vi "Read Props.vi"(8 "error in (no error)":errorcluster, 11 "VerticalSliderControlEditorPanel in":refnum<class "VerticalSliderControlEditorPanel.lvclass">) -> (0 "error out":errorcluster, 2 "Props":T1, 3 "VerticalSliderControlEditorPanel out":refnum<class "VerticalSliderControlEditorPanel.lvclass">)   [LabVIEW 2020, in "VolatusGUIControls.lvlib" / "VerticalSliderControlEditorPanel.lvclass"]
uses:
  VerticalSliderControlEditorPanel.lvclass
  VerticalSliderControlEditorPanel.lvclass/VerticalSliderControlEditorPanel.ctl
  VolatusGUIControls.lvlib
  b4cb06f1-5fc3-472f-9514-749ac11ade19.vi
  JSON Props.ctl
  VolatusGUIEditorCore/VolatusGUIEditorCore.lvlib
  VolatusGUIEditorCore/Label Props.ctl
  VolatusGUIEditorCore/Position Props.ctl
  VolatusGUIEditorCore/Fill Style.ctl
  VolatusGUIEditorCore/Slider Props.ctl
  Props.ctl
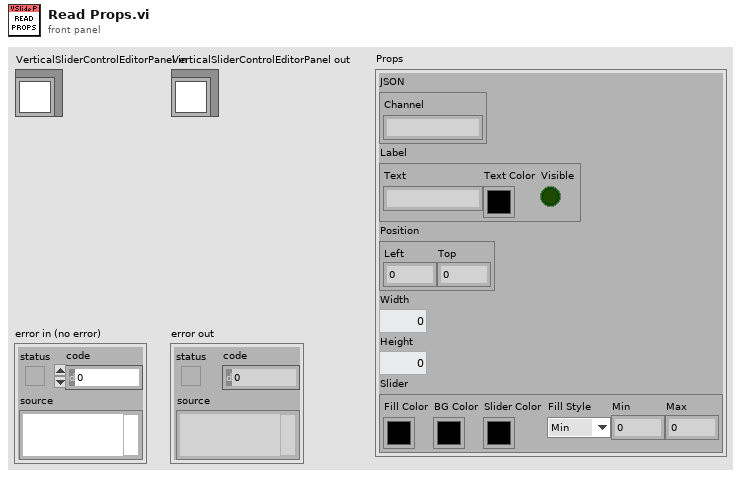
[diagram p1: front panel]
types:
  T1 = typedef "VolatusGUIControls.lvlib/VerticalSliderControlEditorPanel.lvclass/Props.ctl" = cluster{"JSON":T2, "Label":T3, "Position":T4, "Width":u16, "Height":u16, "Slider":T5}
  T2 = typedef "VolatusGUIControls.lvlib/VerticalSliderControlEditorPanel.lvclass/JSON Props.ctl" = cluster{"Channel":string}
  T3 = typedef "VolatusGUIEditorCore.lvlib/Label Props.ctl" = cluster{"Text":string, "Text Color":u32, "Visible":bool}
  T4 = typedef "VolatusGUIEditorCore.lvlib/Position Props.ctl" = cluster{"Left":i32, "Top":i32}
  T5 = typedef "VolatusGUIEditorCore.lvlib/Slider Props.ctl" = cluster{"Fill Color":u32, "BG Color":u32, "Slider Color":u32, "Fill Style":T6, "Min":dbl, "Max":dbl}
  T6 = typedef "VolatusGUIEditorCore.lvlib/Fill Style.ctl" = enum16{"Min", "Max", "None"}
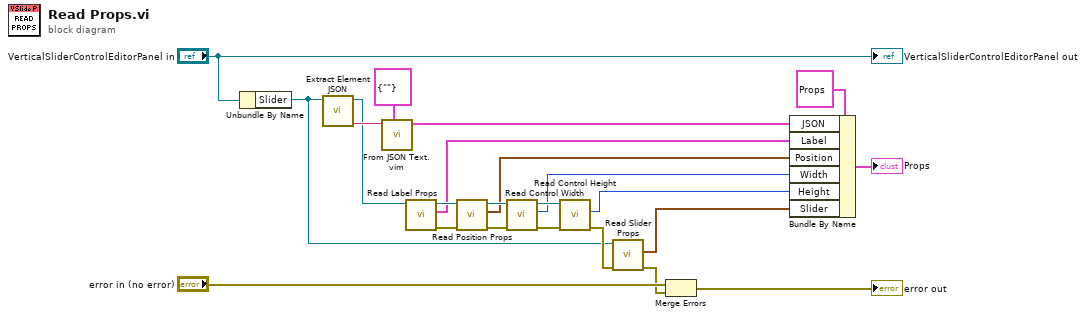
[diagram p0: block diagram]
diagram:
  n1 = Unbundle By Name("VerticalSliderControlEditorPanel in") -> ("Slider"=w11:refnum<vi>)
  n2 = call "Extract Element JSON.vi"("Ctl Refnum in"=w11) -> ("JSON"=w20:string, "Ctl Refnum"=w17:refnum<vi>)  [unwired: 7 in, 2 out]
  n3 = call "From JSON Text.vim"("Data Type and Default Value"=T2 {"Channel"=""} ("JSON Props"), "JSON"=w20) -> ("Data out"=w8:T2)  [unwired: 8 in, 1 out]
  n4 = call "Read Label Props.vi"("Ctl Refnum in"=w17) -> ("error out"=w14:errorcluster, "Label Props"=w7:T3, "Ctl Refnum"=w18:refnum<vi>)  [unwired: 8 in]
  n5 = call "Read Position Props.vi"("error in (no error)"=w14, "Ctl Refnum in"=w18) -> ("error out"=w13:errorcluster, "Position Props"=w6:T4, "Ctl Refnum"=w16:refnum<vi>)  [unwired: 7 in]
  n6 = call "Read Control Width.vi"("error in"=w13, "Control in"=w16) -> ("error out"=w12:errorcluster, "Width"=w5:u32, "Control"=w15:refnum<vi>)  [unwired: 7 in]
  n7 = call "Read Control Height.vi"("error in"=w12, "Control in"=w15) -> ("error out"=w23:errorcluster, "Height"=w4:u32)  [unwired: 7 in, 1 out]
  n8 = call "Read Slider Props.vi"("error in (no error)"=w23, "Slider in"=w11) -> ("error out"=w1:errorcluster, "Slider Props"=w3:T5)  [unwired: 7 in, 1 out]
  n9 = Merge Errors("error in (no error)", w1) -> (→"error out":errorcluster)
  n10 = Bundle By Name(cluster=T1 {"JSON"={"Channel"=""}, "Label"={"Text"="", "Text Color"=0, "Visible"=FALSE}, "Position"={"Left"=0, "Top"=0}, "Width"=0, "Height"=0, "Slider"={"Fill Color"=0, "BG Color"=0, "Slider Color"=0, "Fill Style"=enum."Min", "Min"=0.0, "Max"=0.0}} ("Props"), "JSON"=w8, "Label"=w7, "Position"=w6, "Width"=w5, "Height"=w4, "Slider"=w3) -> (→"Props":T1)
  "VerticalSliderControlEditorPanel out" <- "VerticalSliderControlEditorPanel in"
